vi "set_CurrentBias_subvi.vi"(8 "error in (no error)":errorcluster, 9 "Current":dbl, 10 "Aardvark Handle":i32 min=0, 11 "Address (0x50)":u16=80 max=1023 format="%.0x") -> (0 "error out":errorcluster, 2 "Data Written":bool, 3 "Dup Aardvark Handle":i32)   [LabVIEW 2014]
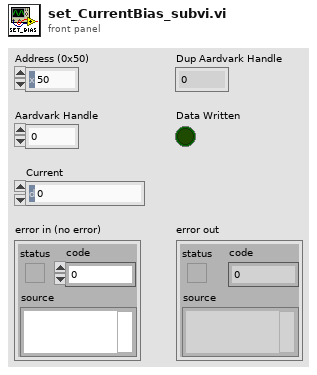
[diagram p1: front panel]
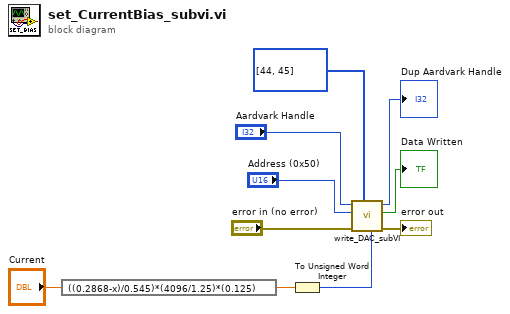
[diagram p0: block diagram]
diagram:
  n1 = expression code="((0.2868-x)/0.545)*(4096/1.25)*(0.125)"("Current") -> (w2:dbl)
  n2 = To Unsigned Word Integer(number=w2) -> (unsigned 16bit integer=w5:u16)
  n3 = call "write_DAC_subVI.vi"("Aardvark Handle in"="Aardvark Handle", "Address (0x50) in"="Address (0x50)", "error in (no error)"="error in (no error)", "DAC_ADD"=u16[] [44, 45], "DAC_Val"=w5) -> ("Dup Aardvark Handle"=→"Dup Aardvark Handle":i32, "DAC Written"=→"Data Written":bool, "error out"=→"error out":errorcluster)  [unwired: 3 in]
